vi "Analog to PWM.vi"() -> ()   [LabVIEW 2026]
panel:
  out "Waveform Chart":u16(graph)
  in  "Pin_AI":u8=4 min=4 max=40
  out "Valor PWM":u8
  in  "Pin_PWM":u8=4 min=4 max=40
  out "Analog read":u16
  in  "VISA resource name":refnum<visa-resource-name>
  in  "Stop Button 2":bool
  # "Demo Analog input - PWM Output"
  # "Convierte la señal analogica (12 bits) a un valor adaptado a la salida de PWM (8 bits)"
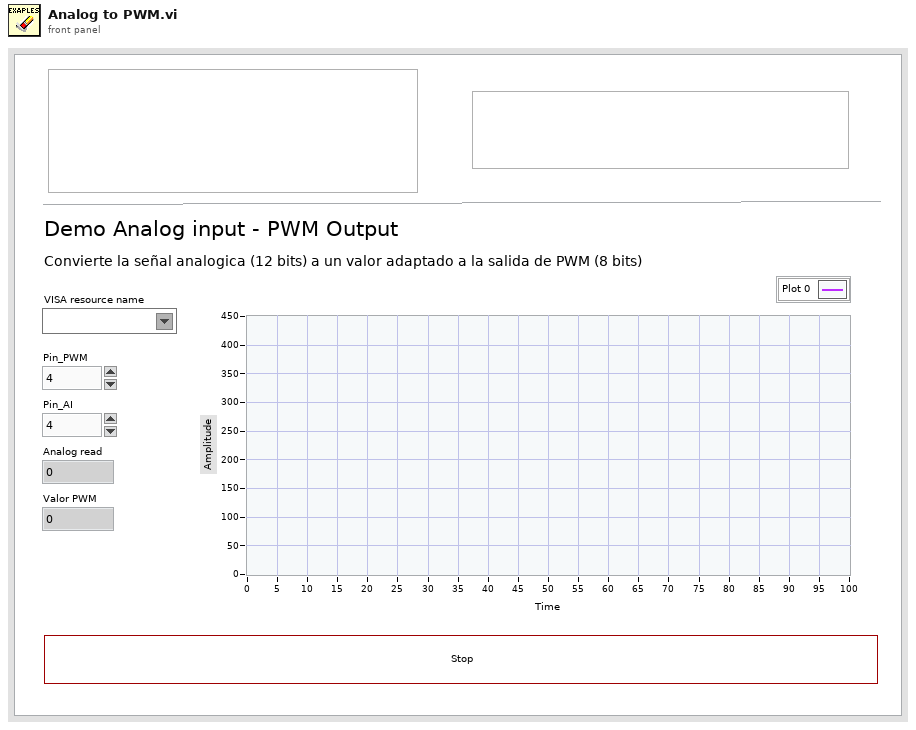
[diagram p1: front panel]
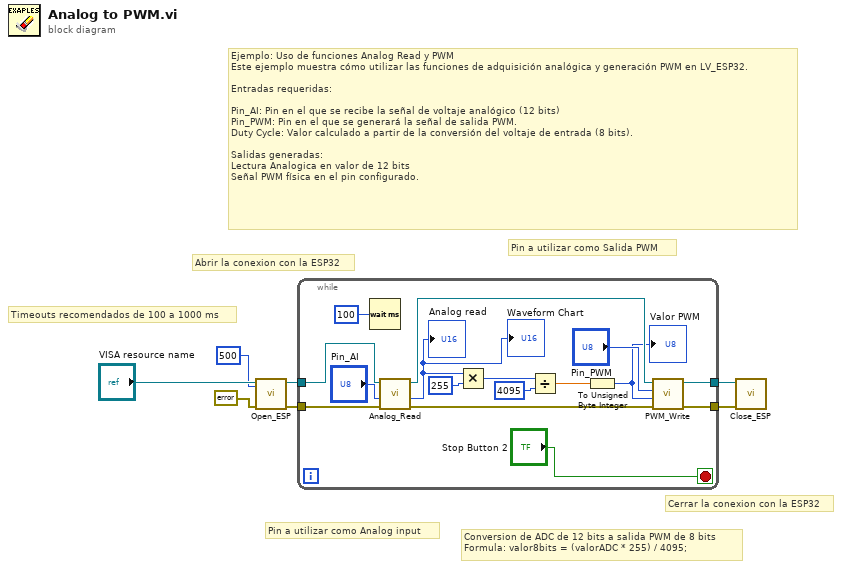
[diagram p0: block diagram]
diagram:
  # "Pin a utilizar como Salida PWM"
  # "Pin a utilizar como Analog input"
  # "Conversion de ADC de 12 bits a salida PWM de 8 bits\nFormula: valor8bits = (valorADC * 255) / 4095;"
  # "Cerrar la conexion con la ESP32"
  # "Timeouts recomendados de 100 a 1000 ms"
  # "Abrir la conexion con la ESP32"
  # "Ejemplo: Uso de funciones Analog Read y PWM\nEste ejemplo muestra cómo utilizar las funciones de adquisición analógica y generación PWM en LV_ESP32.\n\nEntradas requeridas:\n\nPin_AI: Pin en el que se recibe la señal de voltaje analógico (12 bits)\nPin_PWM: Pin en el que se generará la señal de salida PWM.\nDuty Cycle: Valor calculado a partir de la conversión del voltaje de entrada (8 bits).\n\nSalidas generadas:\nLectura Analogica en valor de 12 bits\nSeñal PWM física en el pin configurado."
  n1 = call "Open_ESP.vi"("timeout (10sec)"=u32 500, "error in (no error)"=errorcluster {"status"=FALSE, "code"=0, "source"=""}, "VISA resource name"="VISA resource name") -> ("error out"=w6:errorcluster, "VISA resource name out"=w7:refnum<visa-resource-name>)  [unwired: 7 in]
  n2 = while {
    tunnel: w7 -> [w22]
    tunnel: w6 -> [w23]
    tunnel: [w19] -> w2
    tunnel: [w18] -> w1
    stop <- "Stop Button 2" stop-if-true
    n3 = Wait (ms)(milliseconds to wait=u32 100) -> ()  [unwired: 1 out]
    n4 = call "Analog_Read.vi"("error in (no error)"=w23, "Pin"="Pin_AI", "VISA resource name"=w22) -> ("error out"=w17:errorcluster, "Analog read"=w8:u16, "VISA resource name out"=w20:refnum<visa-resource-name>)  [unwired: 5 in, 1 out]
    "Analog read" <- w8
    "Waveform Chart" <- w8
    n5 = Multiply(x=w8, y=255) -> (x*y=w14:i32)
    n6 = Divide(x=w14, y=4095) -> (x/y=w12:dbl)
    n7 = To Unsigned Byte Integer(number=w12) -> (unsigned 8bit integer=w11:u8)
    "Valor PWM" <- w11
    n8 = call "PWM_Write.vi"("error in (no error)"=w17, "DC"=w11, "Pin"="Pin_PWM", "VISA resource name"=w20) -> ("error out"=w18:errorcluster, "VISA resource name out"=w19:refnum<visa-resource-name>)  [unwired: 6 in]
  }
  n9 = call "Close_ESP.vi"("error in (no error)"=w1, "VISA resource name"=w2) -> ()  [unwired: 9 in, 1 out]
